vi "Get Process List.vi"(6 "Invisible Libraries":string[](array[string]), 8 "Error In":errorcluster, 9 "Remove Library":bool, 11 "Server Name":string="localhost") -> (0 "Error Out":errorcluster, 2 "Libraries":T1, 3 "All Variables":T2)   [LabVIEW 2014]
doc: "<B>Copyright</B>: (c) MHWirth 2015. All rights are reserved.\n\nThis subVI gets the deployed process names and URLs. It can remove those that are specified in \"Invisible Libraries\" from the libraries. Notice the removal does not mean <B>undeployment</B>.\n\nIt also provides all variables info (names + URLs)."
uses:
  <resource>/objmgr/ni.var.rc
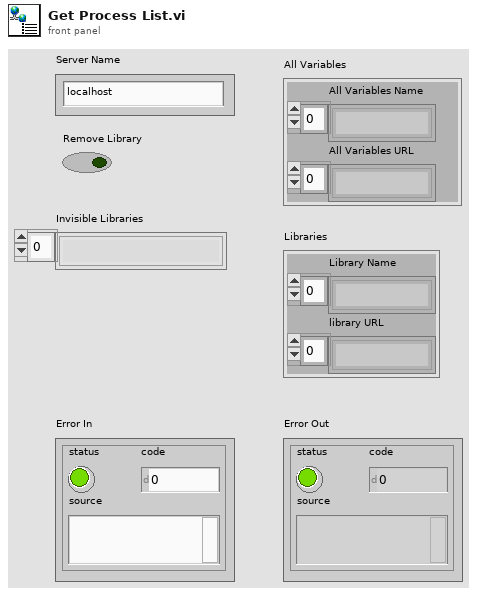
[diagram p1: front panel]
types:
  T1 = cluster{"Library Name":string[], "library URL":string[]}
  T2 = cluster{"All Variables Name":string[], "All Variables URL":string[]}
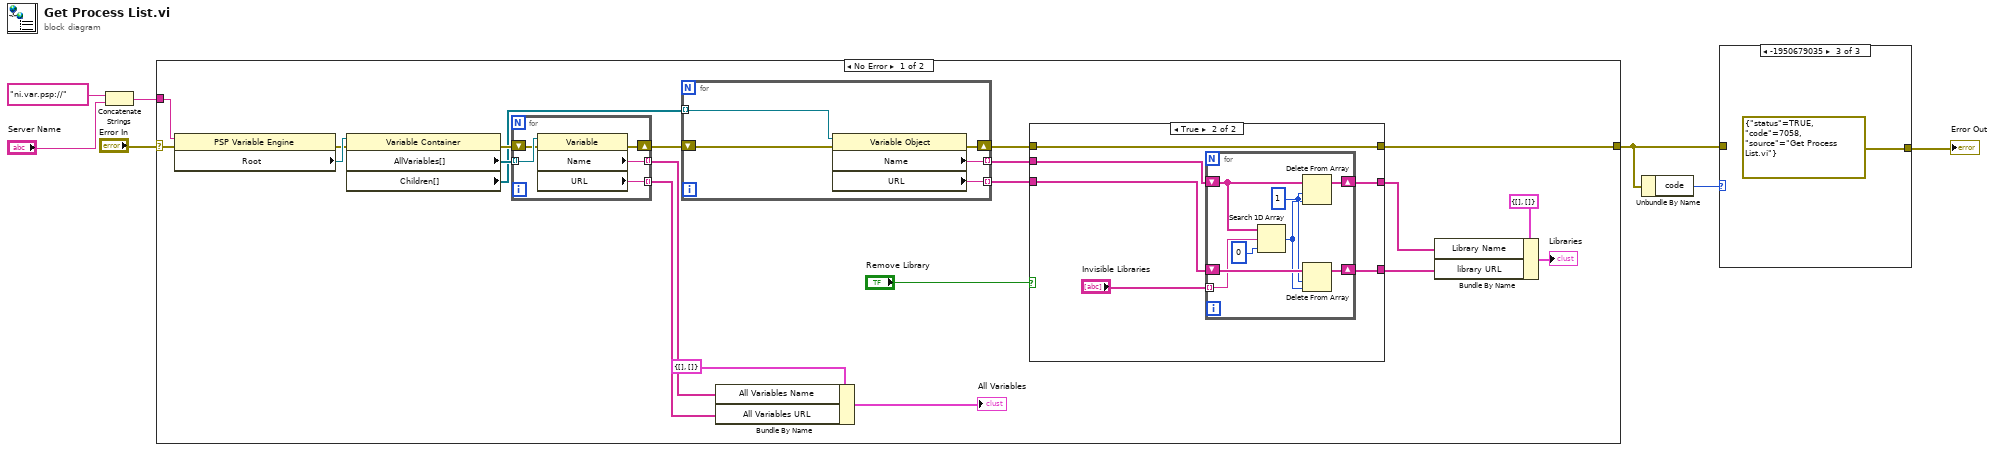
[diagram p0: block diagram]
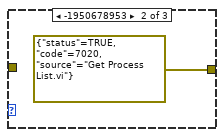
[diagram p3: hidden frame]
diagram:
  n1 = Concatenate Strings("ni.var.psp://", "Server Name") -> (w4:string)
  n2 = case shown="No Error" "Error In" {
    selector: "Error In" -> [w26 w56]
    tunnel: w4 -> [w25 _]
    tunnel: [w8 w56] -> w1
    frame No Error {
      n3 = property class="PSP Variable Engine"(reference=w25, error in=w26) -> (error out=w27:errorcluster, "Root"=w28:refnum<k21>)  [unwired: 1 out]
      n4 = property class="Variable Container"(reference=w28, error in=w27) -> (error out=w23:errorcluster, "AllVariables[]"=w24:refnum<k21>[], "Children[]"=w18:refnum<k21>[])  [unwired: 1 out]
      n5 = for {
        tunnel: w24 -> [w55] mode=indexing
        tunnel: [w54] -> w21 mode=indexing
        tunnel: [w53] -> w20 mode=indexing
        shift-right: [w51] -> w19
        shift-left: w23 -> [w52]
        n6 = property class="Variable"(reference=w55, error in=w52) -> (error out=w51:errorcluster, "Name"=w54:string, "URL"=w53:string)  [unwired: 1 out]
      }
      n7 = for {
        tunnel: w18 -> [w50] mode=indexing
        tunnel: [w49] -> w13 mode=indexing
        tunnel: [w48] -> w12 mode=indexing
        shift-right: [w46] -> w9
        shift-left: w19 -> [w47]
        n8 = property class="Variable Object"(reference=w50, error in=w47) -> (error out=w46:errorcluster, "Name"=w49:string, "URL"=w48:string)  [unwired: 1 out]
      }
      n9 = Bundle By Name(cluster=T2 {"All Variables Name"=[], "All Variables URL"=[]}, "All Variables Name"=w21, "All Variables URL"=w20) -> (→"All Variables":T2)
      n10 = case shown="True" "Remove Library" {
        tunnel: w13 -> [w31 w37]
        tunnel: w12 -> [w30 w36]
        tunnel: [w31 w35] -> w11
        tunnel: [w30 w34] -> w10
        tunnel: [w29 w33] -> w8
        tunnel: w9 -> [w29 w33]
        frame False {
        }
        frame True {
          n11 = for {
            shift-right: [w40] -> w35
            shift-left: w37 -> [w44]
            shift-right: [w39] -> w34
            shift-left: w36 -> [w43]
            tunnel: "Invisible Libraries" -> [w38] mode=indexing
            w42 = 1 ("length")
            n12 = Search 1D Array(1D array=w44, element=w38, start index (0)=0) -> (index of element=w41:i32)
            n13 = Delete From Array(array=w44, length=w42, index=w41) -> (array with subset deleted=w40:string[])  [unwired: 1 out]
            n14 = Delete From Array(array=w43, length=w42, index=w41) -> (array with subset deleted=w39:string[])  [unwired: 1 out]
          }
        }
      }
      n15 = Bundle By Name(cluster=T1 {"Library Name"=[], "library URL"=[]}, "Library Name"=w11, "library URL"=w10) -> (→"Libraries":T1)
    }
    frame Error {
    }
  }
  n16 = Unbundle By Name(w1) -> ("code"=w3:i32)
  n17 = case shown="-1950679035" w3 {
    tunnel: [w57 errorcluster {"status"=TRUE, "code"=7020, "source"="Get Process List.vi"} ("error IO") errorcluster {"status"=TRUE, "code"=7058, "source"="Get Process List.vi"} ("error IO")] -> w2
    tunnel: w1 -> [w57 _ _]
    frame 0, Default {
    }
    frame -1950678953 {
    }
    frame -1950679035 {
    }
  }
  "Error Out" <- w2
